vi "LimeSDR_TwoTone_Tx_LabVIEW_V1.1.vi"() -> ()   [LabVIEW 2018, in "LMS_LV_Drv.lvlib"]
uses:
  LMS_LV_Drv.lvlib
  <vilib>/Analysis/3filter.llb/Filter Passband Type.ctl
  <vilib>/Analysis/NI_AALBase.lvlib
panel:
  out "unsigned 64bit integer":u64=20981760
  out "x/y 2":dbl=20981760.0 format="%#_6f"
  out "size(s) 2":i32=41963520
  out "x/y":dbl=5245440.0
  in  "Boolean":bool
  out "Numeric":i32=77836066
  out "x*y":dbl=20981760.0 format="%#_6f"
  out "size(s)":u64=20981760
  out "return":i32=2098176
  in  "Direction":u8(ring) items=["RX", "TX"]
  out "EXIT":bool=TRUE
  in  "stop":bool
  in  "FM  Frequency":dbl(slide)=500000000.0 min=85000000.0 max=108000000.0 step=50000.0 scale=85000000.0..108000000.0 scale format="%#_6p"
  in  "chan":u64
  out "LimeSDR_info":string="LimeSDR-USB, media=USB 3.0, module=FX3, serial=0009072C02891115, index=0"
  in  "Sample Rate":dbl=2000000.0 format="%#_6p"
  out "error out":errorcluster
  # "Two Tone Generation Demo"
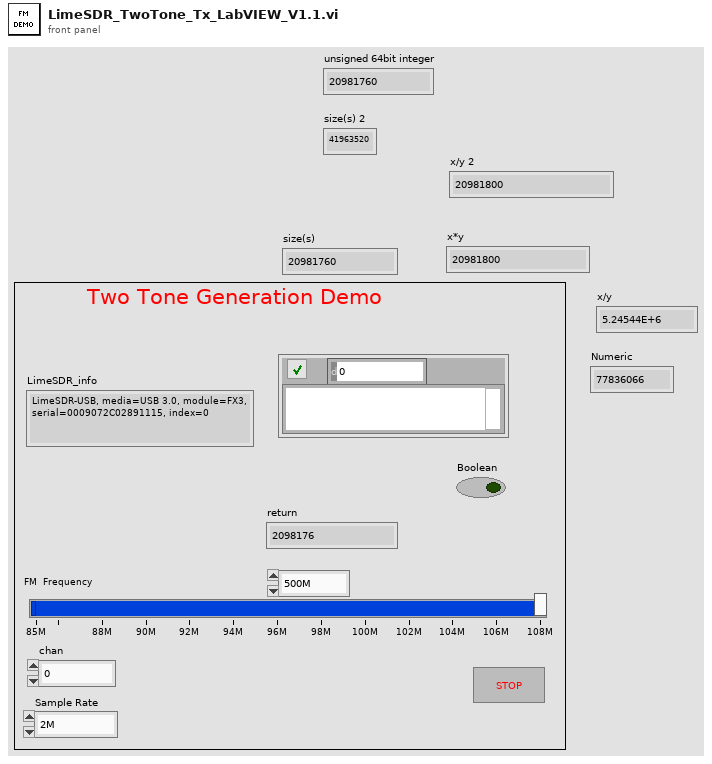
[diagram p1: front panel]
types:
  T1 = typedef "NI_AALBase.lvlib/Filter Passband Type.ctl" = enum32{"Lowpass", "Highpass", "Bandpass", "Bandstop"}
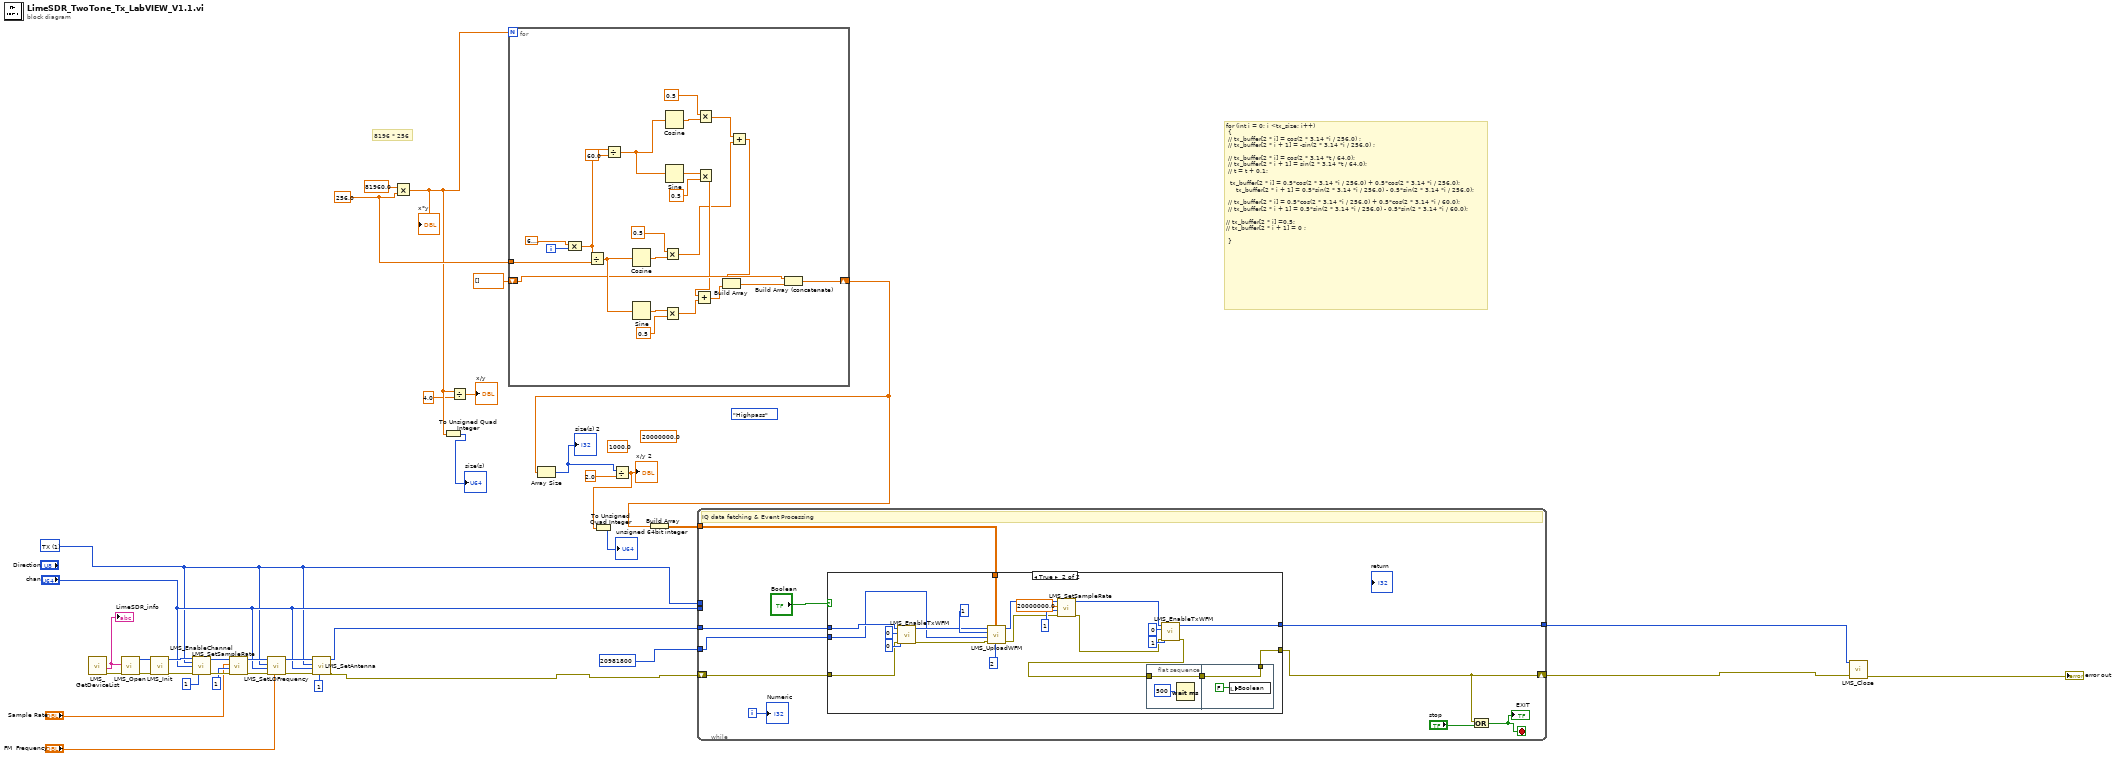
[diagram p0: block diagram]
diagram:
  (unwired) 1000.0 ("low cutoff freq: fl")
  (unwired) 20000000.0 ("sampling freq: fs")
  (unwired) Filter_Passband_Type."Highpass" ("filter type")
  w18 = 256.0 ("x")
  w21 = u8 1 items=["RX", "TX"] ("Direction")
  # "8196 * 256"
  # "for (int i = 0; i <tx_size; i++)\n\t{\n\t//\ttx_buffer[2 * i] = cos(2 * 3.14 *i / 256.0) ;\n\t//\ttx_buffer[2 * i + 1] = -sin(2 * 3.14 *i / 256.0) ;\n\n\t//\ttx_buffer[2 * i] = cos(2 * 3.14 *t / 64.0);\n\t//\ttx_buffer[2 * i + 1] = sin(2 * 3.14 *t / 64.0);\n\t//\tt = t + 0.1;\n\n\t\ttx_buffer[2 * i] = 0.5*cos(2 * 3.14 *i / 256.0) + 0.5*cos(2 * 3.14 *i / 256.0);\n    \ttx_buffer[2 * i + 1] = 0.5*sin(2 * 3.14 *i / 256.0) - 0.5*sin(2 * 3.14 *i / 256.0);\n\n\t//\ttx_buffer[2 * i] = 0.5*cos(2 * 3.14 *i / 256.0) + 0.5*cos(2 * 3.14 *i / 60.0);\n\t//\ttx_buffer[2 * i + 1] = 0.5*sin(2 * 3.14 *i / 256.0) - 0.5*sin(2 * 3.14 *i / 60.0);\n\n//\ttx_buffer[2 * i] =0.5;\n//\ttx_buffer[2 * i + 1] = 0 ;\n\n\t}"
  n1 = call "LMS_GetDeviceList.vi"() -> ("error out"=w38:errorcluster, "lms_info_str_t"=w37:string)  [unwired: 9 in, 1 out]
  "LimeSDR_info" <- w37
  n2 = call "LMS_Open.vi"("error in (no error)"=w38, "lms_info_str_t"=w37) -> ("error out"=w36:errorcluster, "device"=w35:i64)  [unwired: 8 in]
  n3 = call "LMS_Init.vi"("error in (no error)"=w36, "device_In"=w35) -> ("error out"=w33:errorcluster, "device_Out"=w34:i64)  [unwired: 8 in]
  n4 = call "LMS_EnableChannel.vi"("device_In"=w34, "dir_tx"=w21, "chan"="chan", "error in (no error)"=w33, "enabled"=i8 1) -> ("device_Out"=w30:i64, "error out"=w31:errorcluster)  [unwired: 9 in]
  n5 = call "LMS_SetSampleRate.vi"("error in (no error)"=w31, "oversample"=u64 1, "rate"="Sample Rate", "device_In"=w30) -> ("error out"=w29:errorcluster, "device_Out"=w28:i64)  [unwired: 6 in]
  n6 = call "LMS_SetLOFrequency.vi"("frequency"="FM  Frequency", "error in (no error)"=w29, "chan"="chan", "dir_tx"=w21, "device_In"=w28) -> ("error out"=w26:errorcluster, "device_Out"=w25:i64)  [unwired: 5 in]
  n7 = call "LMS_SetAntenna.vi"("index"=u64 1, "error in (no error)"=w26, "chan"="chan", "dir_tx"=w21, "device_In"=w25) -> ("error out"=w15:errorcluster, "device_Out"=w13:i64)  [unwired: 5 in]
  n8 = Multiply(x=81960.0, y=w18) -> (x*y=w9:dbl)
  "x*y" <- w9
  n9 = To Unsigned Quad Integer(1:w9) -> (0:→"size(s)":u64)
  n10 = Divide(x=w9, y=4.0) -> (x/y=→"x/y":dbl)
  n11 = for {
    N: w9 -> [_]
    tunnel: w18 -> [w60]
    shift-right: [w53] -> w10
    shift-left: dbl[] [] -> [w52]
    i -> [w61]
    n12 = Compound Arithmetic op=MULTIPLY(6.283185307179586, w61) -> (w51:dbl)
    n13 = Divide(x=w51, y=w60) -> (x/y=w57:dbl)
    n14 = Divide(x=w51, y=60.0) -> (x/y=w45:dbl)
    n15 = Cosine(x=w57) -> (cos(x)=w59:dbl)
    n16 = Sine(x=w57) -> (sin(x)=w56:dbl)
    n17 = Multiply(x=0.5, y=w59) -> (x*y=w42:dbl)
    n18 = Multiply(x=w56, y=0.5 ("x")) -> (x*y=w41:dbl)
    n19 = Cosine(x=w45) -> (cos(x)=w46:dbl)
    n20 = Sine(x=w45) -> (sin(x)=w48:dbl)
    n21 = Multiply(x=0.5, y=w46) -> (x*y=w44:dbl)
    n22 = Multiply(x=w48, y=0.5 ("x")) -> (x*y=w43:dbl)
    n23 = Add(x=w43, y=w41) -> (x+y=w39:dbl)
    n24 = Add(x=w44, y=w42) -> (x+y=w40:dbl)
    n25 = Build Array(w40, w39) -> (w54:dbl[])
    n26 = Build Array (concatenate)(w52, w54) -> (w53:dbl[])
  }
  n27 = Array Size(array=w10) -> (size(s)=w5:i32)
  "size(s) 2" <- w5
  n28 = Divide(x=w5, y=2.0) -> (x/y=w4:dbl)
  "x/y 2" <- w4
  n29 = To Unsigned Quad Integer(1:w4) -> (0:→"unsigned 64bit integer":u64)
  n30 = Build Array(w10) -> (w11:dbl[][])
  n31 = while {
    shift-right: [w68] -> w14
    shift-left: w15 -> [w69]
    tunnel: w21 -> [_]
    tunnel: "chan" -> [_]
    tunnel: u64 20981800 -> [w64]
    tunnel: w13 -> [w67]
    tunnel: [w66] -> w12
    tunnel: w11 -> [w65]
    i -> [w70]
    stop <- w72 stop-if-true
    # "IQ data fetching & Event Processing"
    n32 = case shown="True" "Boolean" {
      tunnel: w69 -> [w73 w85]
      tunnel: [w73 w90] -> w68
      tunnel: w67 -> [w74 w82]
      tunnel: [w74 w96] -> w66
      tunnel: w65 -> [_ w95]
      tunnel: w64 -> [_ w81]
      frame False {
      }
      frame True {
        n33 = call "LMS_EnableTxWFM.vi"("error in (no error)"=w85, "active"=i8 0, "chan"=u64 0, "device_In"=w82) -> ("error out"=w84:errorcluster, "device_Out"=w83:i64)  [unwired: 6 in]
        n34 = call "LMS_UploadWFM.vi"("format"=2, "samples"=w95, "error in (no error)"=w84, "sample_count"=w81, "ChannelCount"=u8 1, "Dev"=w83) -> ("error out"=w77:errorcluster, "Dev_out"=w79:i64)  [unwired: 4 in]
        n35 = call "LMS_SetSampleRate.vi"("error in (no error)"=w77, "oversample"=u64 1, "rate"=20000000.0, "device_In"=w79) -> ("error out"=w76:errorcluster, "device_Out"=w78:i64)  [unwired: 6 in]
        n36 = flat-sequence {
          tunnel: [w97] -> w89
          tunnel: w88 -> [w97]
          tunnel: [w99] -> w90
          tunnel: w89 -> [w99]
          frame #0 {
            n37 = Wait (ms)(milliseconds to wait=u32 500) -> ()  [unwired: 1 out]
          }
          frame #1 {
            n38 = local write "Boolean"(FALSE ("Boolean")) -> ()
          }
        }
        n39 = call "LMS_EnableTxWFM.vi"("error in (no error)"=w76, "active"=i8 1, "chan"=u64 0, "device_In"=w78) -> ("error out"=w88:errorcluster, "device_Out"=w96:i64)  [unwired: 6 in]
      }
    }
    n40 = Compound Arithmetic op=OR(w68, "stop") -> (w72:bool)
    "EXIT" <- w72
    "Numeric" <- w70
  }
  n41 = call "LMS_Close.vi"("error in (no error)"=w14, "device_In"=w12) -> ("error out"=→"error out":errorcluster)  [unwired: 9 in]
